vi "ReCalcConfig.vi"(0 "Pict Refnum":refnum<vi>, 7 "Image Array":T1[](array[typedef]), 11 "error in (no error)":errorcluster) -> (15 "error out":errorcluster)   [LabVIEW 2013, in "AnimatorXControl.xctl"]
uses:
  AnimatorXControl.xctl
  <vilib>/picture/picture.llb/imagedata.ctl
  DefaultImageData.vi
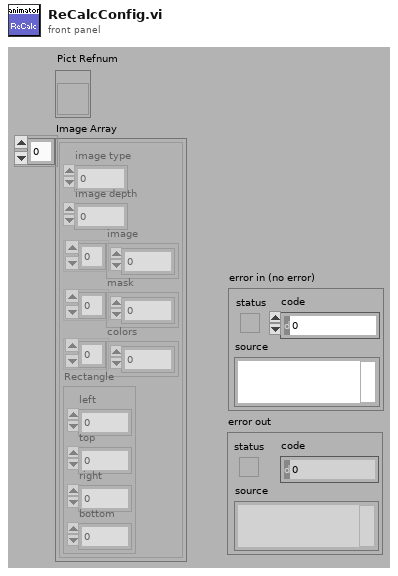
[diagram p1: front panel]
types:
  T1 = typedef "imagedata.ctl" = cluster{"image type":i32, "image depth":i32, "image":u8[], "mask":u8[], "colors":u32[], "Rectangle":cluster{"left":i16, "top":i16, "right":i16, "bottom":i16}}
  T2 = typedef "LVPointTypeDef.ctl" = cluster{"Horizontal":i16, "Vertical":i16}
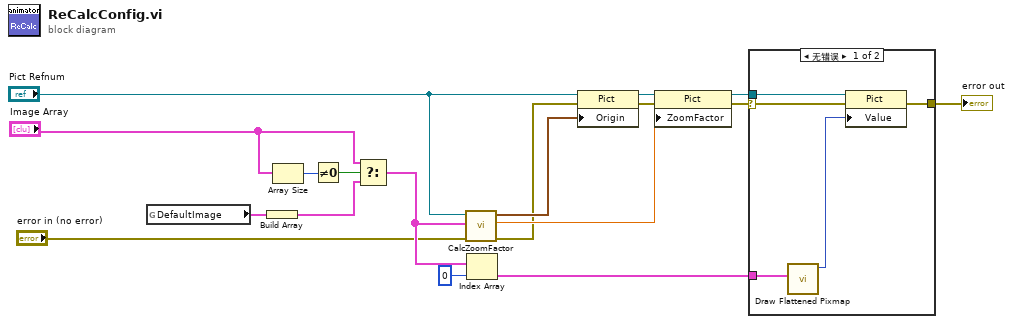
[diagram p0: block diagram]
diagram:
  n1 = global read "DefaultImageData.vi" "DefaultImage"() -> (w17:T1)
  n2 = Build Array(w17) -> (w16:T1[])
  n3 = Array Size(array="Image Array") -> (size(s)=w18:i32)
  n4 = Not Equal To 0?(x=w18) -> (x != 0?=w15:bool)
  n5 = Select(t="Image Array", s=w15, f=w16) -> (s? t:f=w14:T1[])
  n6 = call "CalcZoomFactor.vi"("error in (no error)"="error in (no error)", "Image Array"=w14, "Pict Refnum"="Pict Refnum") -> ("error out"=w6:errorcluster, "ZoomFactor"=w7:dbl, "OriginPoint"=w8:T2)  [unwired: 6 in]
  n7 = Index Array(array=w14, index=0) -> (element=w2:T1)
  n8 = property class="Pict"(reference="Pict Refnum", error in=w6, "Origin"=w8) -> (reference out=w9:refnum<vi>, error out=w5:errorcluster)
  n9 = property class="Pict"(reference=w9, error in=w5, "ZoomFactor"=w7) -> (reference out=w3:refnum<vi>, error out=w4:errorcluster)
  n10 = case shown="无错误" w4 {
    selector: w4 -> [w20 w24]
    tunnel: w3 -> [w22 _]
    tunnel: w2 -> [w23 _]
    tunnel: [w19 w24] -> w1
    frame No Error {
      n11 = call <vilib>:"Draw Flattened Pixmap.vi"("image data"=w23) -> ("new picture"=w21:picture)  [unwired: 8 in]
      n12 = property class="Pict"(reference=w22, error in=w20, "Value"=w21) -> (error out=w19:errorcluster)  [unwired: 1 out]
    }
    frame Error {
    }
  }
  "error out" <- w1
